vi "Get Firmware Name And Version.vi"(8 "error in (no error)":errorcluster, 11 "Transport Parameters in":T1 {"Serial Communication"."Baud Rate" items=["75"=75, "110"=110, "134"=134, "150"=150, "300"=300, "600"=600, "1200"=1200, "1800"=1800, "2400"=2400, "4800"=4800, "7200"=7200, "9600"=9600, "14400"=14400, "19200"=19200, "28800"=28800, "38400"=38400, "56000"=56000, "57600"=57600, "115200"=115200, "128000"=128000, "230400"=230400]}) -> (0 "error out":errorcluster, 1 "FirmataFirmwareVersion":string, 2 "FirmataFirmwareName":string, 3 "Transport Parameters out":T1 {"Serial Communication"."Baud Rate" items=["75"=75, "110"=110, "134"=134, "150"=150, "300"=300, "600"=600, "1200"=1200, "1800"=1800, "2400"=2400, "4800"=4800, "7200"=7200, "9600"=9600, "14400"=14400, "19200"=19200, "28800"=28800, "38400"=38400, "56000"=56000, "57600"=57600, "115200"=115200, "128000"=128000, "230400"=230400]})   [LabVIEW 2020]
uses:
  Controls/ConnectionParameters.ctl
  Controls/SupportedTransports.ctl
  FirmataClient.lvlib
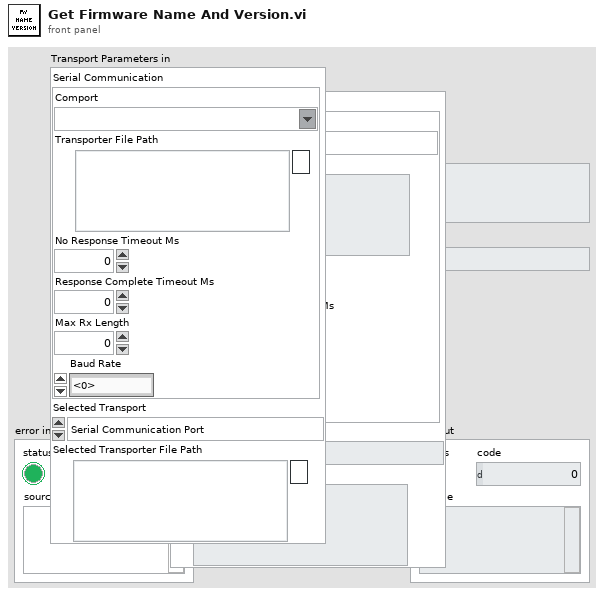
[diagram p1: front panel]
types:
  T1 = typedef "ConnectionParameters.ctl" = cluster{"Serial Communication":cluster{"Comport":refnum<visa-resource-name>, "Transporter File Path":path, "No Response Timeout Ms":u32, "Response Complete Timeout Ms":u32, "Max Rx Length":u32, "Baud Rate":u32}, "Selected Transport":T2, "Selected Transporter File Path":path}
  T2 = typedef "SupportedTransports.ctl" = enum16{"Serial Communication Port"}
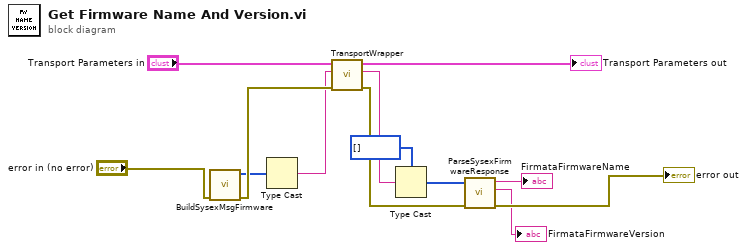
[diagram p0: block diagram]
diagram:
  n1 = call "BuildSysexMsgFirmware.vi"("error in"="error in (no error)") -> ("error out"=w11:errorcluster, "GetFirmwareMessage"=w4:u8[])  [unwired: 7 in, 2 out]
  n2 = Type Cast(x=w4) -> (*(type *) &x=w3:string)  [unwired: 1 in]
  n3 = call "TransportWrapper.vi"("error in"=w11, "Message In"=w3, "Transport Parameters In"="Transport Parameters in") -> ("error out"=w13:errorcluster, "Message Out"=w5:string, "Transport Parameters"=→"Transport Parameters out":T1)  [unwired: 6 in]
  n4 = Type Cast(type=u8[] [] ("GetFirmwareMessage"), x=w5) -> (*(type *) &x=w7:u8[])
  n5 = call "ParseSysexFirmwareResponse.vi"("error in"=w13, "Sysex Message"=w7) -> ("error out"=→"error out":errorcluster, "FirmataFirmwareVersion"=→"FirmataFirmwareVersion":string, "FirmataFirmwareName"=→"FirmataFirmwareName":string)  [unwired: 6 in, 1 out]
